vi "rek.vi"(10 "StringIn":string, 11 "Numeric":i32) -> (2 "StringOut":string)   [LabVIEW 2017]
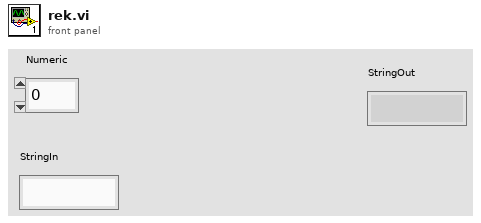
[diagram p1: front panel]
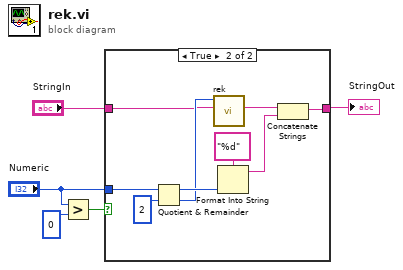
[diagram p0: block diagram]
diagram:
  n1 = Greater?(x="Numeric", y=0) -> (0:w4:bool)
  n2 = case shown="True" w4 {
    tunnel: "Numeric" -> [_ w12]
    tunnel: [w6 w10] -> w1
    tunnel: "StringIn" -> [w6 w8]
    frame False {
    }
    frame True {
      n3 = Quotient & Remainder(x=w12, y=2) -> (x-y*floor(x/y)=w13:i32, floor(x/y)=w11:i32)
      n4 = call "rek.vi"("StringIn"=w8, "Numeric"=w11) -> ("StringOut"=w7:string)  [unwired: 9 in]
      n5 = Format Into String(format string="%d", w13) -> (resulting string=w9:string)  [unwired: 2 in, 1 out]
      n6 = Concatenate Strings(w7, w9) -> (w10:string)
    }
  }
  "StringOut" <- w1
